vi "Visor_ondas.vi"() -> ()   [LabVIEW 2026]
uses:
  <vilib>/Math Plots/3D Math Plots/3D Pie/3D Pie XCtrl/3D Pie.xctl
  <vilib>/Utility/file.llb/Read Delimited Spreadsheet (string).vi
  <vilib>/Math Plots/3D Math Plots/3D Pie/3D Pie Datatype/Public/Plot Helper (Vector).vi
  <vilib>/Math Plots/3D Math Plots/3D Pie/3D Pie Datatype/3D Pie Datatype.lvclass
panel:
  out "3D Pie":refnum<class "3D Plot Datatype.lvclass">[](xcontrol)
  out "B":i32
  out "G":i32
  out "R":i32
  out "Colores":digitalwaveform[](graph)
  out "Status":digitalwaveform[](graph)
  in  "Leer CSV":bool
  in  "stop":bool
  out "all rows":string[][](array[string])
  in  "Archivo CSV":path
  # "ocN = 1 el motor N esta ocupado"
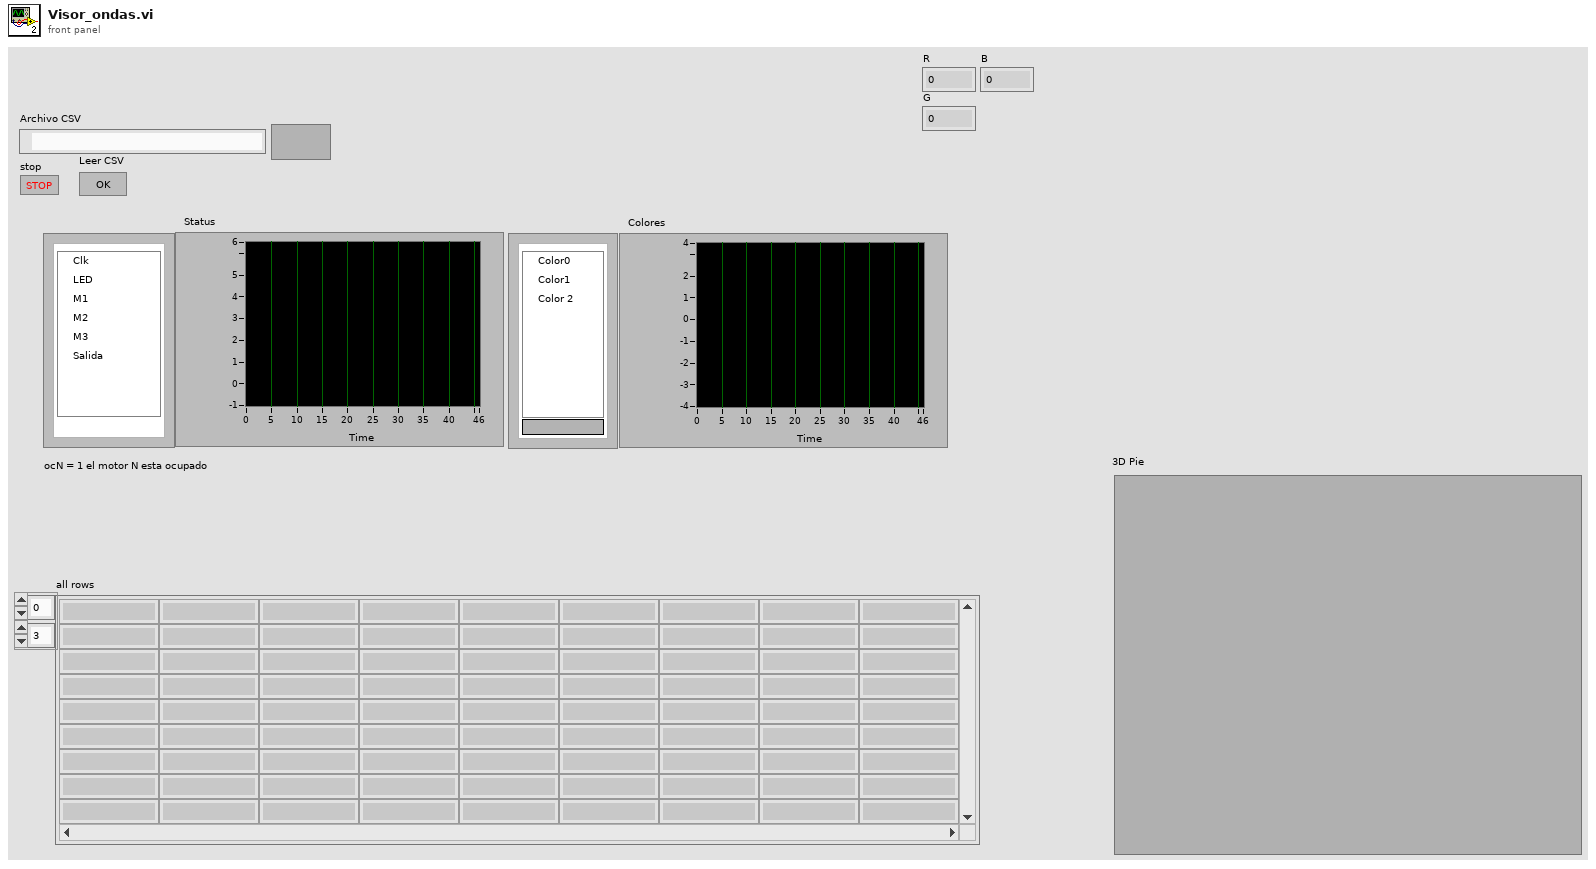
[diagram p1: front panel]
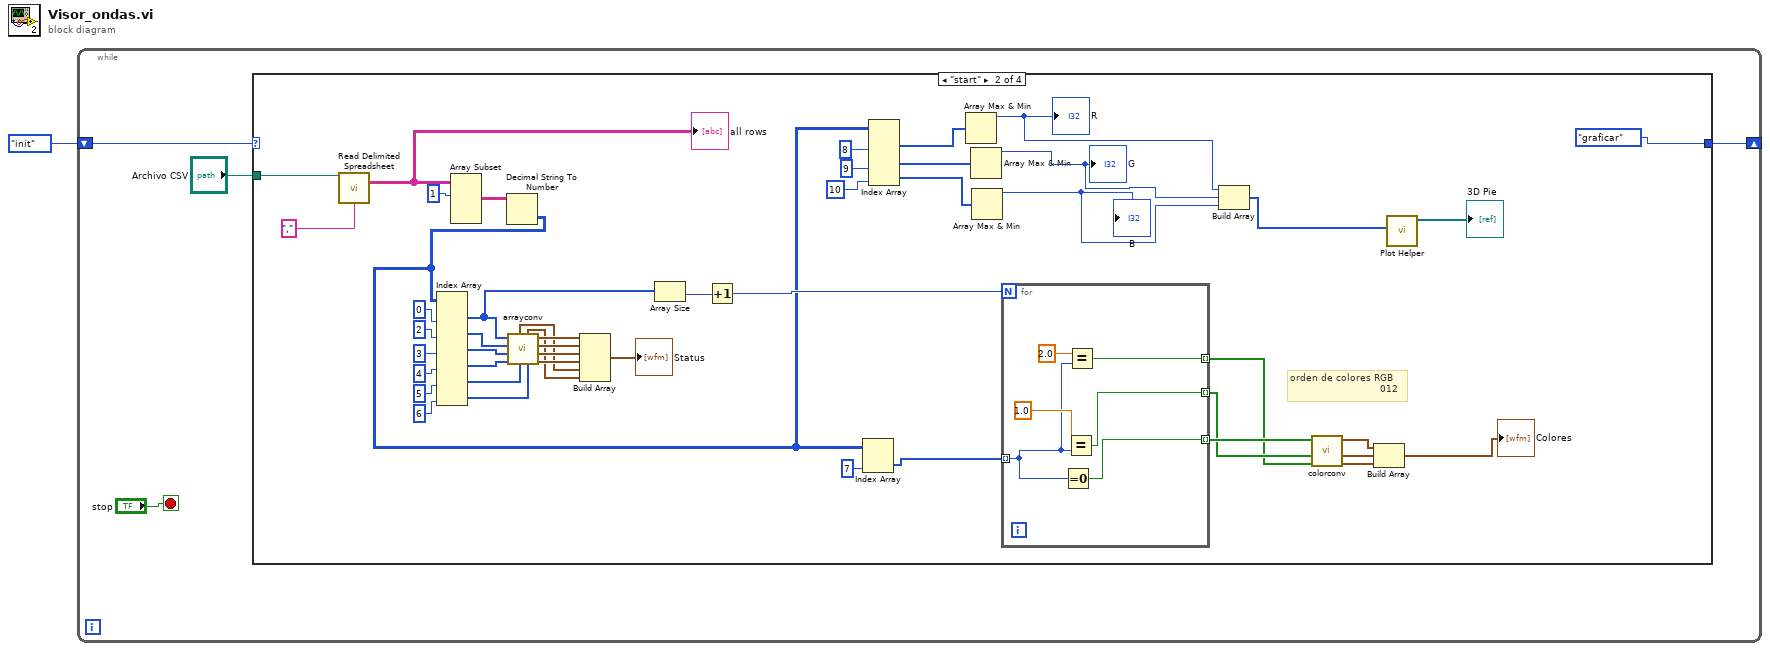
[diagram p0: block diagram]
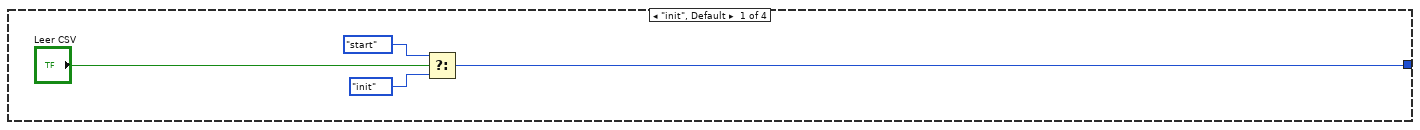
[diagram p2: hidden frame]
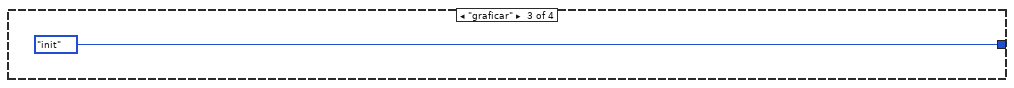
[diagram p3: hidden frame]
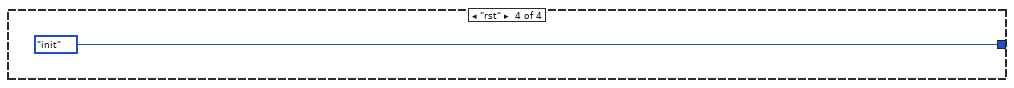
[diagram p4: hidden frame]
diagram:
  n1 = while {
    shift-right: [w2] -> _
    shift-left: enum16{"init", "start", "graficar", "rst"}."init" -> [w3]
    stop <- "stop" stop-if-true
    n2 = case shown="\"start\"" w3 {
      tunnel: "Archivo CSV" -> [_ w56 _ _]
      tunnel: [w6 enum16{"init", "start", "graficar", "rst"}."graficar" enum16{"init", "start", "graficar", "rst"}."init" enum16{"init", "start", "graficar", "rst"}."init"] -> w2
      frame "init", Default {
        n3 = Select(t=enum16{"init", "start", "graficar", "rst"}."start", s="Leer CSV", f=enum16{"init", "start", "graficar", "rst"}."init") -> (s? t:f=w6:enum16{"init", "start", "graficar", "rst"})
      }
      frame "start" {
        # "orden de colores RGB \n                              012"
        n4 = call-poly <vilib>:"Read Delimited Spreadsheet.vi"("file path (dialog if empty)"=w56, "delimiter (\\t)"="," ("delimiter (\\t)")) -> ("all rows"=w54:string[][])  [unwired: 8 in, 5 out]
        "all rows" <- w54
        n5 = Array Subset(array=w54, index (row)=1 ("index")) -> (w52:string[][])  [unwired: 3 in]
        n6 = Decimal String To Number(string=w52) -> (number=w21:i32[][])  [unwired: 2 in, 1 out]
        n7 = Index Array(array=w21, index (col) #1=0 ("disabled index (col)"), index (col) #2=2 ("disabled index (col)"), index (col) #3=3 ("disabled index (col)"), index (col) #4=4 ("disabled index (col)"), index (col) #5=5 ("disabled index (col)"), index (col) #6=6 ("index (col)")) -> (element #1=w32:i32[], element #2=w46:i32[], element #3=w45:i32[], element #4=w44:i32[], element #5=w43:i32[], element #6=w35:i32[])  [unwired: 6 in]
        n8 = call "arrayconv.vi"("Input 6"=w35, "Input 5"=w43, "Input 4"=w44, "Input 3"=w45, "Input 2"=w46, "Input 1"=w32) -> ("output waveform 4"=w39:digitalwaveform, "output waveform 3"=w40:digitalwaveform, "output waveform 2"=w41:digitalwaveform, "output waveform"=w42:digitalwaveform, "output waveform 6"=w34:digitalwaveform, "output waveform 5"=w38:digitalwaveform)
        n9 = Build Array(w42, w41, w40, w39, w38, w34) -> (→"Status":digitalwaveform[])
        n10 = Array Size(array=w32) -> (size(s)=w31:i32)
        n11 = Increment(x=w31) -> (x+1=w30:i32)
        n12 = Index Array(array=w21, index (col)=7 ("disabled index (col)")) -> (element=w29:i32[])  [unwired: 1 in]
        n13 = Index Array(array=w21, index (col) #1=8 ("disabled index (col)"), index (col) #2=9 ("disabled index (col)"), index (col) #3=10 ("disabled index (col)")) -> (element #1=w17:i32[], element #2=w15:i32[], element #3=w16:i32[])  [unwired: 3 in]
        n14 = Array Max & Min(array=w17) -> (max value=w13:i32)  [unwired: 3 out]
        "R" <- w13
        n15 = Array Max & Min(array=w15) -> (max value=w12:i32)  [unwired: 3 out]
        "G" <- w12
        n16 = Array Max & Min(array=w16) -> (max value=w11:i32)  [unwired: 3 out]
        "B" <- w11
        n17 = for {
          N: w30 -> [_]
          tunnel: w29 -> [w59] mode=indexing
          tunnel: [w62] -> w27 mode=indexing
          tunnel: [w61] -> w28 mode=indexing
          tunnel: [w58] -> w26 mode=indexing
          n18 = Equal To 0?(x=w59) -> (x = 0?=w61:bool)
          n19 = Equal?(x=1.0, y=w59) -> (x = y?=w62:bool)
          n20 = Equal?(x=2.0, y=w59) -> (x = y?=w58:bool)
        }
        n21 = Build Array(w13, w12, w11) -> (w10:i32[])
        n22 = call "colorconv.vi"("Color 3"=w26, "Color 2"=w27, "Color 1"=w28) -> ("output waveform 3"=w23:digitalwaveform, "output waveform 2"=w24:digitalwaveform, "output waveform"=w25:digitalwaveform)  [unwired: 6 in]
        n23 = Build Array(w25, w24, w23) -> (→"Colores":digitalwaveform[])
        n24 = call-poly <vilib>:"Plot Helper.vi"("x vector"=w10) -> ("3D Plot lvclass Array out"=→"3D Pie":refnum<class "3D Plot Datatype.lvclass">[])  [unwired: 2 in, 8 out]
      }
      frame "graficar" {
      }
      frame "rst" {
      }
    }
  }
